vi "TSM Set DAQmx AI Tasks.vi"(0 "TSM context":T1, 5 "Sampling Rate (Hz)":dbl format="%#_6pHz", 7 "Samples per channel":i32=1000, 9 "Range (V)":dbl=3.0, 11 "error in (no error)":errorcluster) -> (15 "error out":errorcluster)   [LabVIEW 2020]
doc: "Use this VI to initialize AI and AO tasks for all NI-DAQmx instruments in the pin map associated with the test program."
uses:
  <vilib>/NI_TestStand_SemiconductorModule/NI_TestStand_Semiconductor_Module.lvlibp/PinMap/General/SemiconductorModuleContext.ctl
  <vilib>/DAQmx/create/channels.llb/DAQmx Create Channel (AI-Voltage-Basic).vi
  <vilib>/DAQmx/configure/timing.llb/DAQmx Timing (Sample Clock).vi
  <vilib>/NI_TestStand_SemiconductorModule/NI_TestStand_Semiconductor_Module.lvlibp
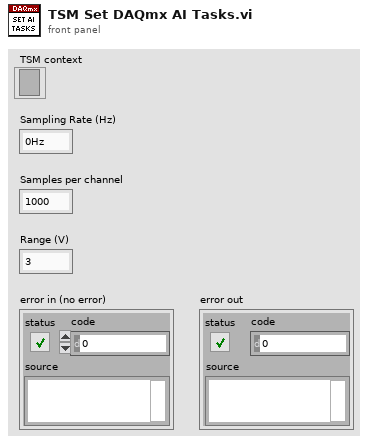
[diagram p1: front panel]
types:
  T1 = typedef "NI_TestStand_Semiconductor_Module.lvlibp/SemiconductorModuleContext.ctl" = refnum<k7>
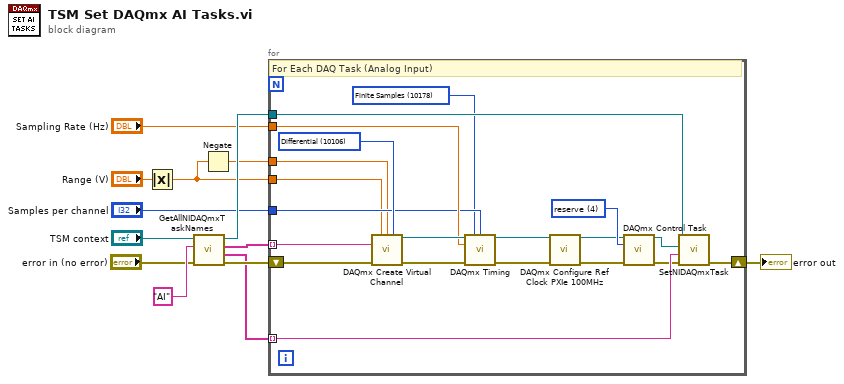
[diagram p0: block diagram]
diagram:
  n1 = Absolute Value(x="Range (V)") -> (abs(x)=w2:dbl)
  n2 = call <vilib>:"GetAllNIDAQmxTaskNames.vi"("error in (no error)"="error in (no error)", "Task Type"="AI", "Semiconductor Module Context"="TSM context") -> ("error out"=w12:errorcluster, "Task Names"=w11:string[], "Channel Lists"=w10:string[], "Semiconductor Module Context Out"=w13:T1)  [unwired: 5 in]
  n3 = Negate(x=w2) -> (-x=w3:dbl)
  n4 = for {
    tunnel: w13 -> [w32]
    tunnel: w11 -> [w28] mode=indexing
    tunnel: w10 -> [w30] mode=indexing
    shift-right: [w31] -> w5
    shift-left: w12 -> [w33]
    tunnel: "Sampling Rate (Hz)" -> [w25]
    tunnel: "Samples per channel" -> [w24]
    tunnel: w2 -> [w14]
    tunnel: w3 -> [w15]
    w22 = 4 items=["verify"=2, "reserve"=4, "commit"=3, "unreserve"=5, "abort"=6] ("action")
    w23 = 10178 items=["Finite Samples"=10178, "Continuous Samples"=10123, "Hardware Timed Single Point"=12522] ("sample mode")
    w29 = 10106 items=["default"=-1, "RSE"=10083, "NRSE"=10078, "Differential"=10106, "Pseudodifferential"=12529] ("input terminal configuration")
    # "For Each DAQ Task (Analog Input)"
    n5 = call-poly <vilib>:"DAQmx Create Virtual Channel.vi"("maximum value"=w14, "minimum value"=w15, "input terminal configuration"=w29, "physical channels"=w30, "error in"=w33) -> ("task out"=w26:refnum<k21>, "error out"=w27:errorcluster)  [unwired: 9 in]
    n6 = call-poly <vilib>:"DAQmx Timing.vi"("task/channels in"=w26, "sample mode"=w23, "samples per channel"=w24, "rate"=w25, "error in"=w27) -> ("task out"=w19:refnum<k21>, "error out"=w18:errorcluster)  [unwired: 9 in]
    n7 = call "DAQmx Configure Ref Clock PXIe 100MHz.vi"("DAQmx Task In"=w19, "error in (no error)"=w18) -> ("DAQmx Task Out"=w17:refnum<k21>, "error out"=w16:errorcluster)  [unwired: 12 in]
    n8 = call <vilib>:"DAQmx Control Task.vi"("task/channels in"=w17, "action"=w22, "error in"=w16) -> ("task out"=w21:refnum<k21>, "error out"=w20:errorcluster)  [unwired: 11 in]
    n9 = call <vilib>:"SetNIDAQmxTask.vi"("error in (no error)"=w20, "Task Name"=w28, "DAQmx Task"=w21, "Semiconductor Module Context"=w32) -> ("error out"=w31:errorcluster)  [unwired: 6 in, 1 out]
  }
  "error out" <- w5
